vi "ViPER_Dialog.vi"() -> ()   [LabVIEW 2022 SP3]
uses:
  <vilib>/Utility/config.llb/Read Key (String).vi
  <vilib>/Utility/config.llb/Write Key (String).vi
  <vilib>/Utility/config.llb/NI_LVConfig.lvlib
panel:
  in  "Abort":bool
  in  "Start":bool
  in  "Name":string caption="String"
  in  "Path":path
  # "Build ViPER Component"
  # "ViPER Component"
  # ".net"
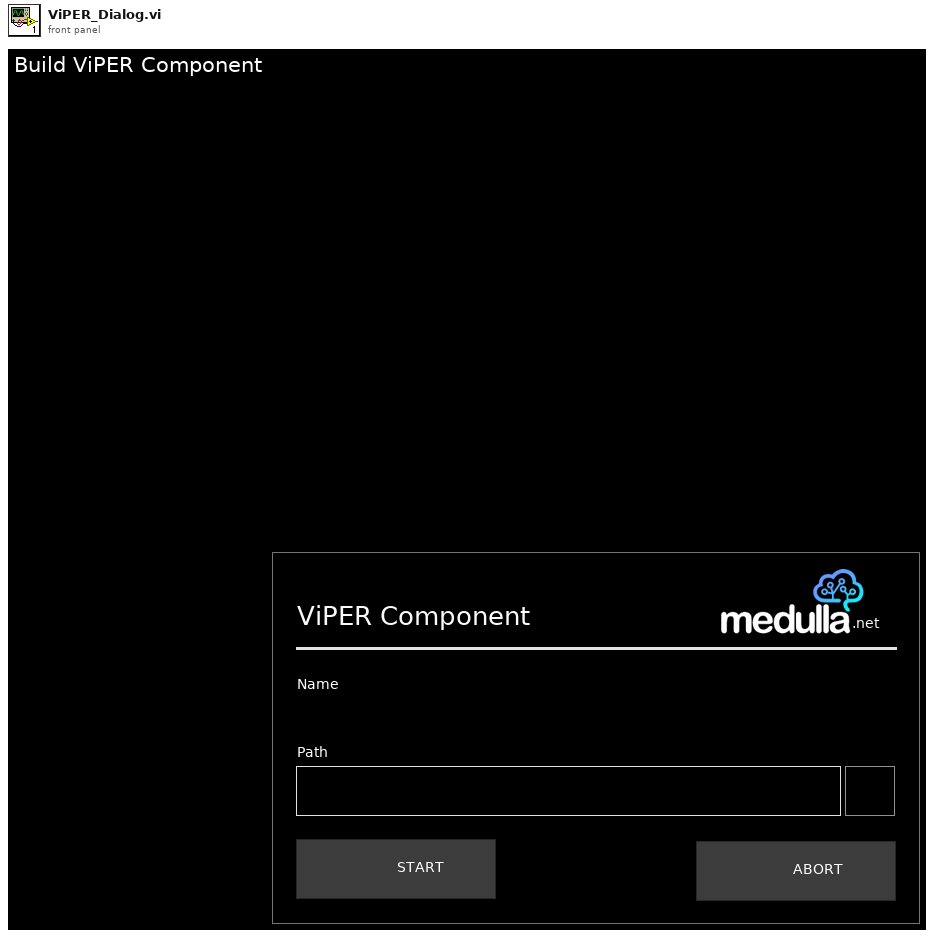
[diagram p1: front panel]
types:
  T1 = enum32{"Invalid", "Standard", "Closed", "Hidden", "Minimized", "Maximized"}
  T2 = enum8{"Enabled", "Disabled", "Disabled and Grayed Out"}
  T3 = typedef "NI_LVConfig.lvlib/Config Data RefNum.ctl" = refnum<k1>
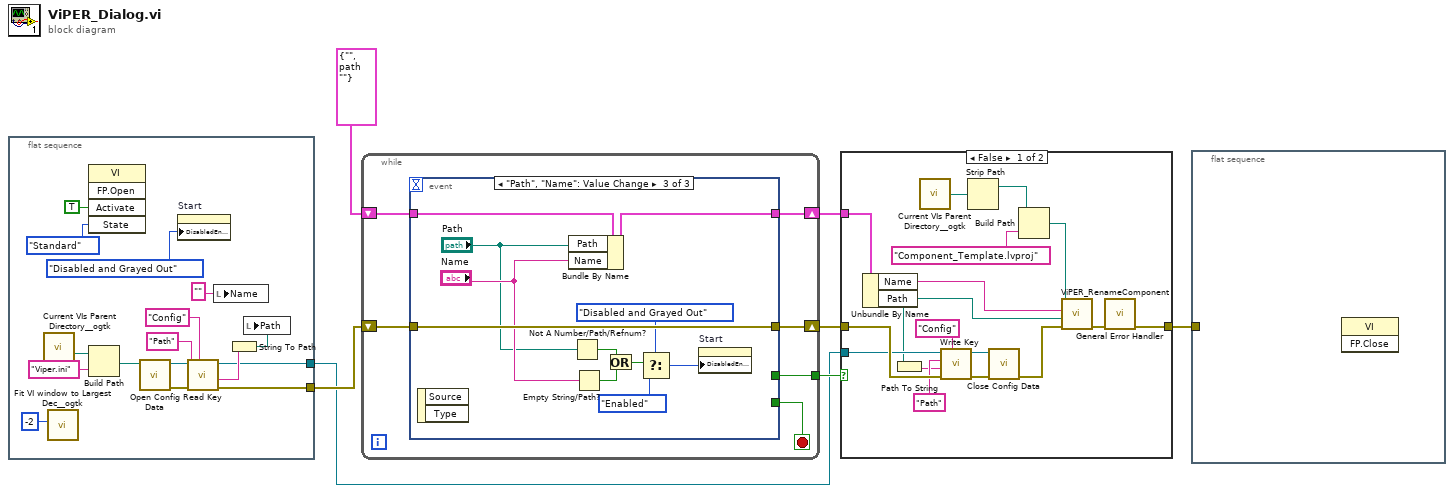
[diagram p0: block diagram]
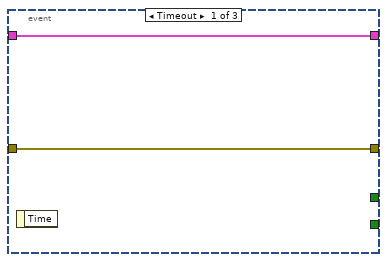
[diagram p3: hidden frame]
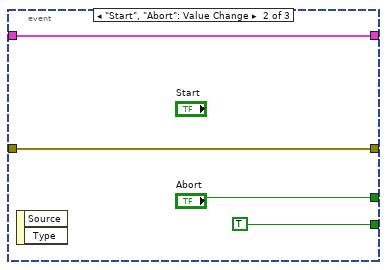
[diagram p4: hidden frame]
diagram:
  n1 = flat-sequence {
    tunnel: [w13] -> w7
    tunnel: [w8] -> w2
    frame #0 {
      n2 = call <userlib>:"Current VIs Parent Directory__ogtk.vi"() -> ("Parent Directory (+ Relative)"=w18:path)  [unwired: 5 in]
      n3 = call <userlib>:"Fit VI window to Largest Dec__ogtk.vi"("border spacing (2 px)"=-2) -> ()  [unwired: 5 in, 2 out]
      n4 = invoke class="VI" method="FP.Open"("Activate"=TRUE ("Activate?"), "State"=T1."Standard") -> ()  [unwired: 3 in, 5 out]
      n5 = Build Path(base path=w18, name or relative path="Viper.ini") -> (appended path=w16:path)
      n6 = call <vilib>:"Open Config Data.vi"("configuration file path"=w16) -> ("error out"=w14:errorcluster, "refnum"=w15:T3)  [unwired: 8 in, 1 out]
      n7 = property on="Start" class="Bool (strict)"("DisabledEnum"=T2."Disabled and Grayed Out" ("Disabled")) -> ()  [unwired: 2 in, 2 out]
      n8 = call-poly <vilib>:"Read Key.vi"("section"="Config", "error in (no error)"=w14, "key"="Path", "refnum"=w15) -> ("error out"=w13:errorcluster, "value"=w10:string, "refnum out"=w8:T3)  [unwired: 4 in, 1 out]
      n9 = local write "Name"("" ("Name")) -> ()
      n10 = String To Path(string=w10) -> (path=w9:path)
      n11 = local write "Path"(w9) -> ()
    }
  }
  n12 = while {
    shift-right: [w26] -> w4
    shift-left: w7 -> [w29]
    tunnel: [w27] -> w6
    shift-right: [w24] -> w3
    shift-left: cluster{"Name":string, "Path":path} {"Name"="", "Path"=path ""} -> [w25]
    stop <- w28 stop-if-true
    n13 = event shown="[2] \"Path\", \"Name\": Value Change" {
      selector: _ -> [_ _ _]
      dyn-events: _ -> [_ _ _]
      timeout: _ -> [_ _ _]
      tunnel: w29 -> [w31 w32 w46]
      tunnel: [_ TRUE ("OK") _] -> w28
      tunnel: [_ "Abort" _] -> w27
      tunnel: [w31 w32 w46] -> w26
      tunnel: w25 -> [w30 w34 w45]
      tunnel: [w30 w34 w44] -> w24
      event Timeout {
        n14 = event-data() -> ()  [unwired: 1 in, 1 out]
      }
      event "Start", "Abort": Value Change {
        n15 = event-data() -> ()  [unwired: 1 in, 2 out]
      }
      event "Path", "Name": Value Change {
        n16 = event-data() -> ()  [unwired: 1 in, 2 out]
        n17 = Bundle By Name(cluster=w45, "Path"="Path", "Name"="Name") -> (w44:cluster{"Name":string, "Path":path})
        n18 = Not A Number/Path/Refnum?(number/path/refnum="Path") -> (NaN/Path/Refnum?=w43:bool)
        n19 = Empty String/Path?(string/path="Name") -> (empty?=w42:bool)
        n20 = Or(x=w43, y=w42) -> (x .or. y?=w41:bool)
        n21 = Select(t=T2."Disabled and Grayed Out" ("Disabled"), s=w41, f=T2."Enabled" ("Disabled")) -> (s? t:f=w37:T2)
        n22 = property on="Start" class="Bool (strict)"("DisabledEnum"=w37) -> ()  [unwired: 2 in, 2 out]
      }
    }
  }
  n23 = case shown="False" w6 {
    tunnel: w4 -> [w56 _]
    tunnel: w3 -> [w63 _]
    tunnel: w2 -> [w55 _]
    tunnel: [w47 _] -> w1
    frame False {
      n24 = Unbundle By Name(w63) -> ("Name"=w62:string, "Path"=w49:path)
      n25 = Path To String(path=w49) -> (string=w48:string)
      n26 = call <userlib>:"Current VIs Parent Directory__ogtk.vi"() -> ("Parent Directory (+ Relative)"=w61:path)  [unwired: 5 in]
      n27 = call-poly <vilib>:"Write Key.vi"("section"="Config", "error in (no error)"=w56, "value"=w48, "key"="Path", "refnum"=w55) -> ("error out"=w54:errorcluster, "refnum out"=w52:T3)  [unwired: 4 in, 1 out]
      n28 = Strip Path(path=w61) -> (stripped path=w60:path)  [unwired: 1 out]
      n29 = call <vilib>:"Close Config Data.vi"("error in (no error)"=w54, "refnum"=w52) -> ("error out"=w53:errorcluster)  [unwired: 8 in, 1 out]
      n30 = Build Path(base path=w60, name or relative path="Component_Template.lvproj") -> (appended path=w58:path)
      n31 = call "ViPER_RenameComponent.vi"("error in (no error)"=w53, "Target Path"=w49, "Component Name"=w62, "ComponentTemplate"=w58) -> ("error out"=w57:errorcluster)  [unwired: 7 in]
      n32 = call <vilib>:"General Error Handler.vi"("error in (no error)"=w57) -> ("error out"=w47:errorcluster)  [unwired: 10 in, 4 out]
    }
    frame True {
    }
  }
  n33 = flat-sequence {
    tunnel: w1 -> [_]
    frame #0 {
      n34 = invoke class="VI" method="FP.Close"() -> ()  [unwired: 3 in, 3 out]
    }
  }
